vi "Write Digital Outputs.vi"(8 "error in (no error)":errorcluster, 11 "PXI6521 in":refnum<class "PXI6521.lvclass">) -> (0 "error out":errorcluster, 3 "PXI6521 out":refnum<class "PXI6521.lvclass">)   [LabVIEW 2018, in "PXI6521.lvlib" / "PXI6521.lvclass"]
uses:
  PXI6521.lvclass
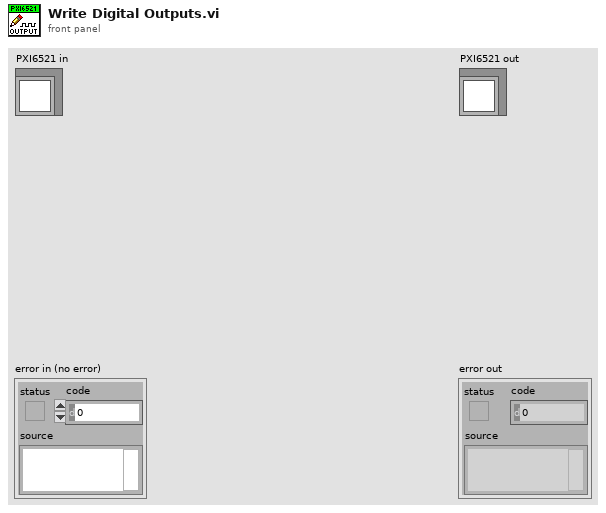
[diagram p1: front panel]
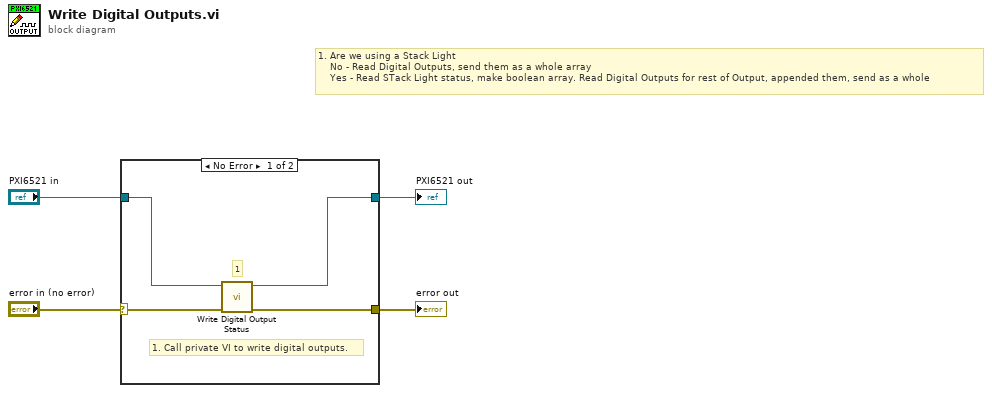
[diagram p0: block diagram]
diagram:
  # "1. Are we using a Stack Light\n    No - Read Digital Outputs, send them as a whole array\n    Yes - Read STack Light status, make boolean array. Read Digital Outputs for rest of Output, appended them, send as a whole"
  n1 = case shown="No Error" "error in (no error)" {
    selector: "error in (no error)" -> [w8 w10]
    tunnel: [w5 w10] -> w3
    tunnel: [w6 w9] -> w2
    tunnel: "PXI6521 in" -> [w7 w9]
    frame No Error {
      # "1. Call private VI to write digital outputs."
      # "1"
      n2 = call "Write Digital Output Status.vi"("error in (no error)"=w8, "PXI6521 in"=w7) -> ("error out"=w5:errorcluster, "PXI6521 out"=w6:refnum<class "PXI6521.lvclass">)  [unwired: 8 in]
    }
    frame Error {
    }
  }
  "error out" <- w3
  "PXI6521 out" <- w2
